vi "failure to error cluster.vi"(8 "failure":T1 {"code" format="%.0x"}) -> (0 "error in":errorcluster)   [LabVIEW 2013]
uses:
  failure.ctl
  const sourcename.vi
  get message.vi
  get default message.vi
  const messagename.vi
  <vilib>/Utility/error.llb/Error Code Database.vi
  failure.lvlib
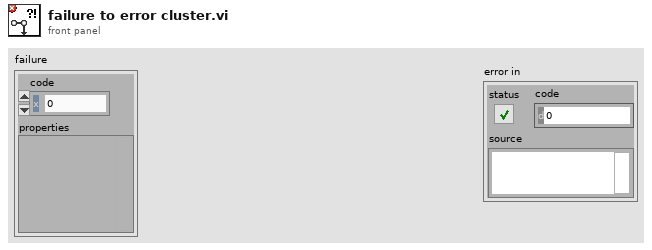
[diagram p1: front panel]
types:
  T1 = typedef "failure.lvlib/failure.ctl" = cluster{"code":i32, "properties":variant}
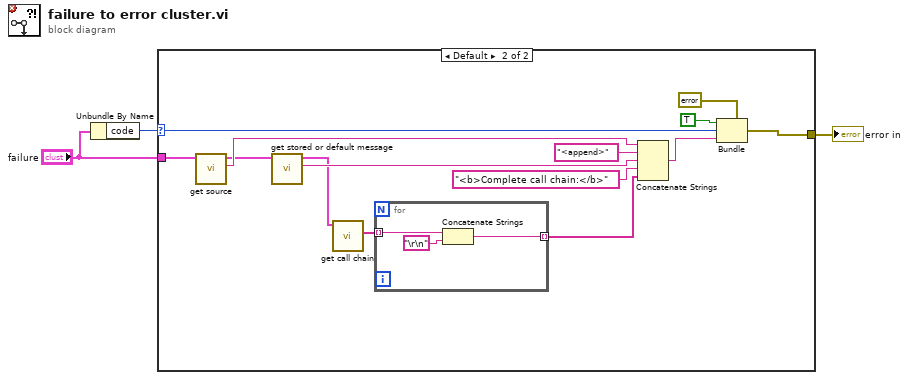
[diagram p0: block diagram]
diagram:
  n1 = Unbundle By Name("failure") -> ("code"=w2:i32)
  n2 = case shown="Default" w2 {
    selector: w2 -> [_ w16]
    tunnel: [_ w17] -> w3
    tunnel: "failure" -> [_ w15]
    frame 0 {
    }
    frame Default {
      n3 = call "get source.vi"("failure in"=w15) -> ("source"=w13:string, "failure out"=w9:T1)  [unwired: 9 in]
      n4 = call "get stored or default message.vi"("failure in"=w9) -> ("message"=w8:string, "failure out"=w6:T1)  [unwired: 9 in]
      n5 = call "get call chain.vi"("failure in"=w6) -> ("call chain"=w5:string[])  [unwired: 9 in, 1 out]
      n6 = for {
        tunnel: w5 -> [w20] mode=indexing
        tunnel: [w19] -> w4 mode=indexing
        n7 = Concatenate Strings(w20, "\r\n") -> (w19:string)
      }
      n8 = Concatenate Strings(w13, "<append>" ("string"), w8, "<b>Complete call chain:</b>" ("string"), w4) -> (w11:string)
      n9 = Bundle(cluster=errorcluster {"status"=FALSE, "code"=0, "source"=""} ("error in 2"), "status"=TRUE, "code"=w16, "source"=w11) -> (w17:errorcluster)
    }
  }
  "error in" <- w3
